vi "modify 2 servo 12.vi"() -> ()   [LabVIEW 2012]
uses:
  <vilib>/Motion/FlexMotion/FunctionsVIs/AxisResourceConfig.llb/Enable Axes (8 axes).flx
  <vilib>/Motion/FlexMotion/FunctionsVIs/Trajectory.llb/Load Accel/Decel in RPS/sec.flx
  <vilib>/Motion/FlexMotion/FunctionsVIs/StartStopMotion.llb/Start Motion (8 axes).flx
  <vilib>/Motion/FlexMotion/FunctionsVIs/Trajectory.llb/Check Move Complete Status (8 axes).flx
  <vilib>/Motion/FlexMotion/FunctionsVIs/StartStopMotion.llb/Stop Motion (8 axes).flx
panel:
  in  "RUN":bool
  out "indicated vel":dbl=-499.7589111328125
  in  "STOP":bool
  in  "VELOCITY in RPM":dbl=500.0
  in  "CHANGE DIRECTION":bool
  in  "acceleration(rps/s)":dbl=1000.0 format="%.2f"
  in  "CHOOSE AXIS":T1
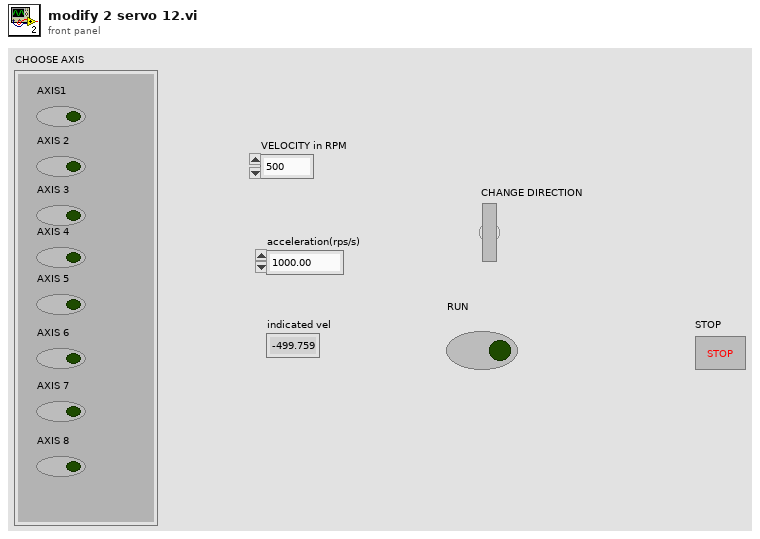
[diagram p1: front panel]
types:
  T1 = cluster{"AXIS1":bool, "AXIS 2":bool, "AXIS 3":bool, "AXIS 4":bool, "AXIS 5":bool, "AXIS 6":bool, "AXIS 7":bool, "AXIS 8":bool}
  T2 = enum16{"Absolute Position", "Relative Position", "Velocity", "Relative to Cap Pos", "Modulus Position", "Absolute Contouring", "Relative Contouring"}
  T3 = typedef "Board Id" = u8
  T4 = typedef "Resource Out (Enum).flx" = u16
  T5 = typedef "Bd Id Out" = u8
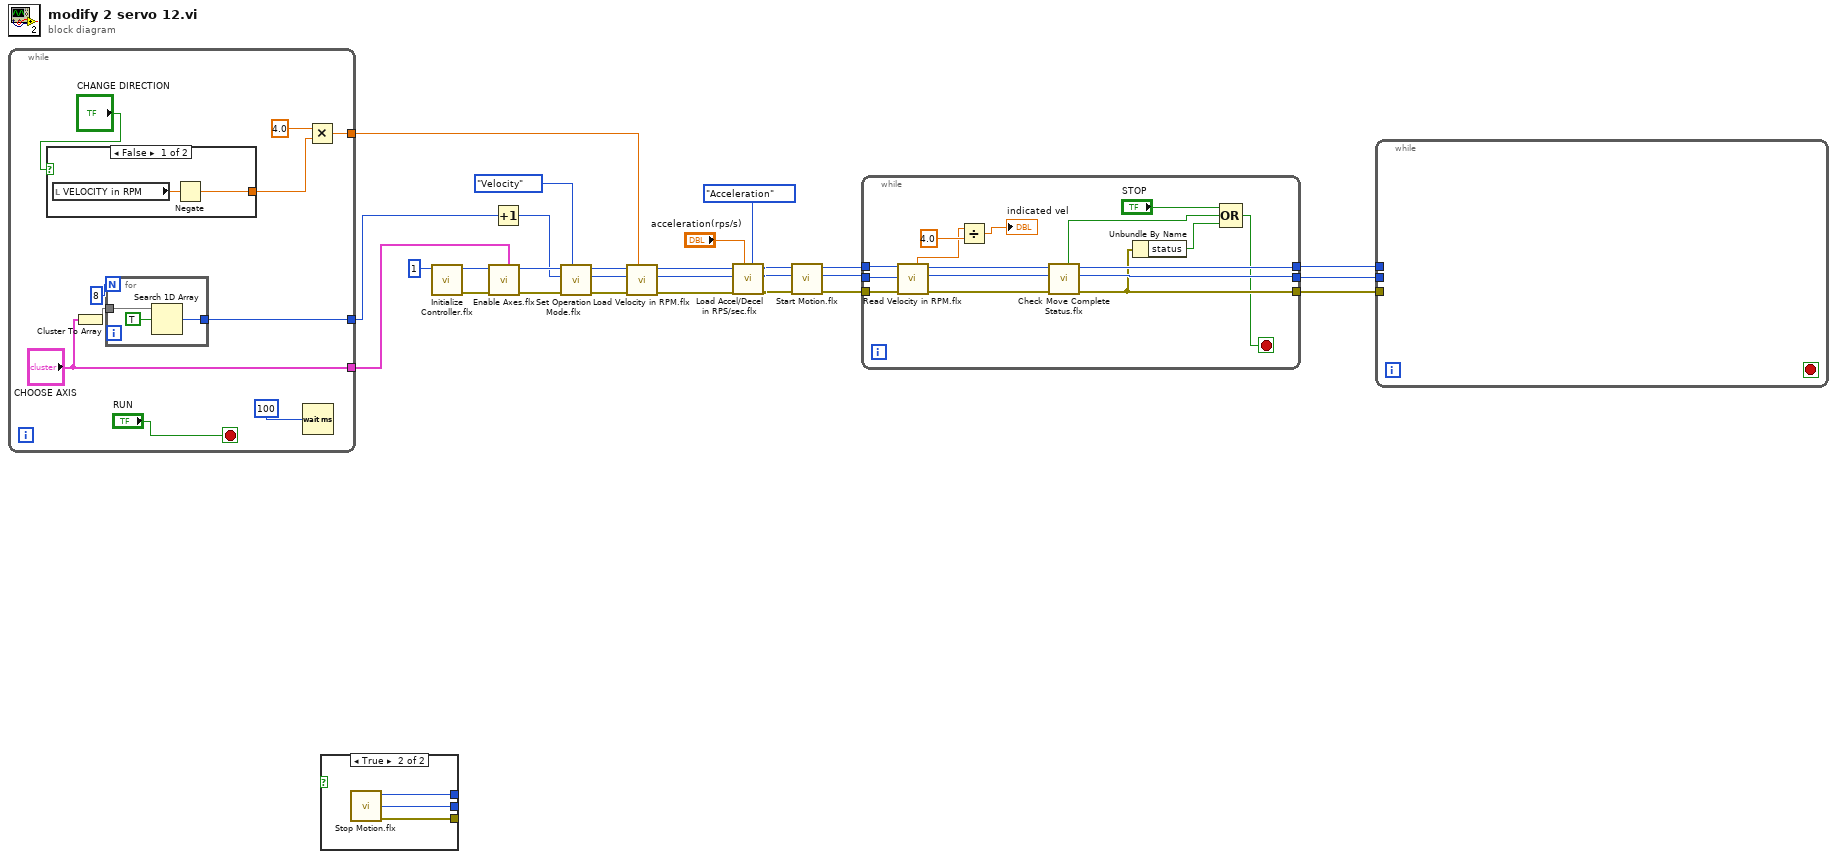
[diagram p0: block diagram]
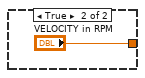
[diagram p3: hidden frame]
diagram:
  n1 = while {
    tunnel: ["CHOOSE AXIS"] -> w21
    tunnel: [w35] -> w20
    tunnel: [w29] -> w5
    stop <- "RUN" stop-if-true
    n2 = case shown="False" "CHANGE DIRECTION" {
      tunnel: [w38 "VELOCITY in RPM"] -> w30
      frame False {
        n3 = local read "VELOCITY in RPM"() -> (w39:dbl)
        n4 = Negate(x=w39) -> (-x=w38:dbl)
      }
      frame True {
      }
    }
    n5 = Cluster To Array(cluster="CHOOSE AXIS") -> (array=w36:bool[])
    n6 = for {
      N: 8 -> [_]
      tunnel: w36 -> [w43]
      tunnel: [w41] -> w35
      n7 = Search 1D Array(1D array=w43, element=TRUE) -> (index of element=w41:i32)  [unwired: 1 in]
    }
    n8 = Wait (ms)(milliseconds to wait=u32 100) -> ()  [unwired: 1 out]
    n9 = Multiply(x=4.0 ("y"), y=w30) -> (x*y=w29:dbl)
  }
  n10 = case shown="True" {
    selector: _ -> [_ _]
    tunnel: [_ w46] -> _
    tunnel: [_ w45] -> _
    tunnel: [_ w44] -> _
    frame False {
    }
    frame True {
      n11 = call-poly <vilib>:"Stop Motion.flx"() -> ("error out"=w46:errorcluster, "Resource Output"=w44:T4, "Bd ID Out"=w45:T5)  [unwired: 7 in]
    }
  }
  n12 = call <vilib>:"Initialize Controller.flx"("Board ID"=T3 1) -> ("error out"=w25:errorcluster, "Bd ID Out"=w26:T5)  [unwired: 7 in]
  n13 = call-poly <vilib>:"Enable Axes.flx"("Axis Bitmap (Disabled)"=w21, "error in (no error)"=w25, "Board ID"=w26) -> ("error out"=w24:errorcluster, "Bd ID Out"=w23:T5)  [unwired: 5 in]
  n14 = Increment(x=w20) -> (x+1=w1:i32)
  n15 = call <vilib>:"Set Operation Mode.flx"("Position Mode (Absolute)"=T2."Velocity", "error in (no error)"=w24, "Axis or Vector Space"=w1, "Board ID"=w23) -> ("error out"=w7:errorcluster, "Resource Output"=w8:T4, "Bd ID Out"=w9:T5)  [unwired: 2 in]
  n16 = call <vilib>:"Load Velocity in RPM.flx"("Velocity (500)"=w5, "error in (no error)"=w7, "Axis or Vector Space"=w8, "Board ID"=w9) -> ("error out"=w16:errorcluster, "Resource Output"=w17:T4, "Bd ID Out"=w18:T5)  [unwired: 3 in]
  n17 = call "Load Accel/Decel in RPS/sec.flx"("Selector (Both)"=enum16{"Both", "Acceleration", "Deceleration"}."Acceleration", "Value (200)"="acceleration(rps/s)", "error in (no error)"=w16, "Axis or Vector Space"=w17, "Board ID"=w18) -> ("error out"=w10:errorcluster, "Resource Output"=w11:T4, "Bd ID Out"=w12:T5)  [unwired: 2 in]
  n18 = call-poly <vilib>:"Start Motion.flx"("error in (no error)"=w10, "Axis or Vector Space"=w11, "Board ID"=w12) -> ("error out"=w15:errorcluster, "Resource Output"=w14:T4, "Bd ID Out"=w13:T5)  [unwired: 3 in]
  n19 = while {
    tunnel: [w62] -> w4
    tunnel: [w61] -> w3
    tunnel: [w60] -> w2
    tunnel: w15 -> [w55]
    tunnel: w14 -> [w54]
    tunnel: w13 -> [w53]
    stop <- w52 stop-if-true
    n20 = call <vilib>:"Read Velocity in RPM.flx"("error in (no error)"=w55, "Axis or Vector Space"=w54, "Board ID"=w53) -> ("error out"=w57:errorcluster, "Resource Output"=w58:T4, "Bd ID Out"=w59:T5, "Filtered Velocity"=w50:dbl)  [unwired: 3 in]
    n21 = Divide(x=w50, y=4.0) -> (x/y=→"indicated vel":dbl)
    n22 = call-poly <vilib>:"Check Move Complete Status.flx"("error in (no error)"=w57, "Axis or Vector Space"=w58, "Board ID"=w59) -> ("error out"=w60:errorcluster, "Resource Output"=w61:T4, "Bd ID Out"=w62:T5, "Move Complete"=w48:bool)  [unwired: 3 in]
    n23 = Unbundle By Name(w60) -> ("status"=w49:bool)
    n24 = Compound Arithmetic op=OR("STOP", w48, w49) -> (w52:bool)
  }
  n25 = while {
    tunnel: w4 -> [_]
    tunnel: w3 -> [_]
    tunnel: w2 -> [_]
    stop <- _ stop-if-true
  }
